vi "matrix.vi"(2 "B":T2, 3 "A":T3) -> (0 "P":T1, 1 "X0":bool)   [LabVIEW 2013]
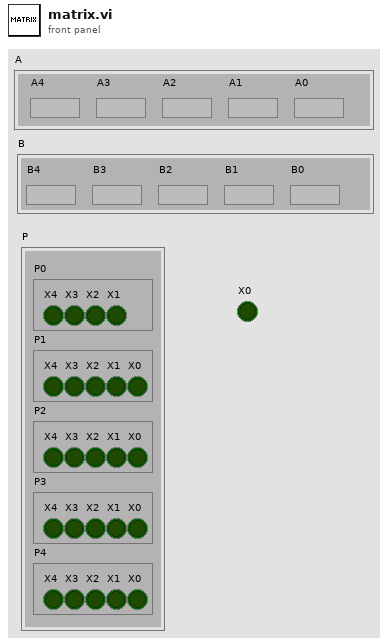
[diagram p1: front panel]
types:
  T1 = cluster{"P0":cluster{"X4":bool, "X3":bool, "X2":bool, "X1":bool}, "P1":cluster{"X4":bool, "X3":bool, "X2":bool, "X1":bool, "X0":bool}, "P2":cluster{"X4":bool, "X3":bool, "X2":bool, "X1":bool, "X0":bool}, "P3":cluster{"X4":bool, "X3":bool, "X2":bool, "X1":bool, "X0":bool}, "P4":cluster{"X4":bool, "X3":bool, "X2":bool, "X1":bool, "X0":bool}}
  T2 = cluster{"B4":bool, "B3":bool, "B2":bool, "B1":bool, "B0":bool}
  T3 = cluster{"A4":bool, "A3":bool, "A2":bool, "A1":bool, "A0":bool}
  T4 = cluster{cluster{bool, bool, bool, bool}, cluster{bool, bool, bool, bool, bool}, cluster{bool, bool, bool, bool, bool}, cluster{bool, bool, bool, bool, bool}, cluster{bool, bool, bool, bool, bool}}
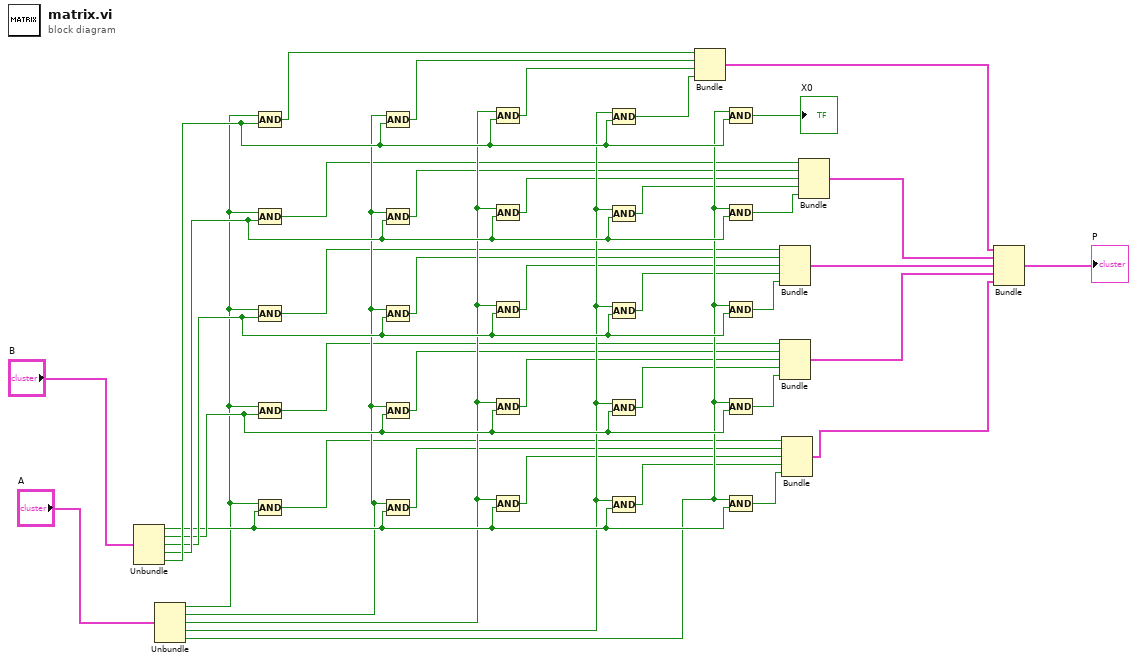
[diagram p0: block diagram]
diagram:
  n1 = Unbundle("B") -> ("B4"=w37:bool, "B3"=w38:bool, "B2"=w39:bool, "B1"=w40:bool, "B0"=w41:bool)
  n2 = Unbundle("A") -> ("A4"=w32:bool, "A3"=w33:bool, "A2"=w34:bool, "A1"=w35:bool, "A0"=w36:bool)
  n3 = Compound Arithmetic op=AND(w32, w41) -> (w27:bool)
  n4 = Compound Arithmetic op=AND(w32, w40) -> (w22:bool)
  n5 = Compound Arithmetic op=AND(w32, w39) -> (w17:bool)
  n6 = Compound Arithmetic op=AND(w32, w38) -> (w12:bool)
  n7 = Compound Arithmetic op=AND(w32, w37) -> (w7:bool)
  n8 = Compound Arithmetic op=AND(w33, w41) -> (w28:bool)
  n9 = Compound Arithmetic op=AND(w33, w40) -> (w23:bool)
  n10 = Compound Arithmetic op=AND(w33, w39) -> (w18:bool)
  n11 = Compound Arithmetic op=AND(w33, w38) -> (w13:bool)
  n12 = Compound Arithmetic op=AND(w33, w37) -> (w8:bool)
  n13 = Compound Arithmetic op=AND(w34, w41) -> (w29:bool)
  n14 = Compound Arithmetic op=AND(w34, w40) -> (w24:bool)
  n15 = Compound Arithmetic op=AND(w34, w39) -> (w19:bool)
  n16 = Compound Arithmetic op=AND(w34, w38) -> (w14:bool)
  n17 = Compound Arithmetic op=AND(w34, w37) -> (w9:bool)
  n18 = Compound Arithmetic op=AND(w35, w41) -> (w30:bool)
  n19 = Compound Arithmetic op=AND(w35, w40) -> (w25:bool)
  n20 = Compound Arithmetic op=AND(w35, w39) -> (w20:bool)
  n21 = Compound Arithmetic op=AND(w35, w38) -> (w15:bool)
  n22 = Compound Arithmetic op=AND(w35, w37) -> (w10:bool)
  n23 = Bundle(w27, w28, w29, w30) -> (w5:cluster{bool, bool, bool, bool})  [unwired: 1 in]
  n24 = Compound Arithmetic op=AND(w36, w41) -> (→"X0":bool)
  n25 = Compound Arithmetic op=AND(w36, w40) -> (w26:bool)
  n26 = Compound Arithmetic op=AND(w36, w39) -> (w21:bool)
  n27 = Compound Arithmetic op=AND(w36, w38) -> (w16:bool)
  n28 = Compound Arithmetic op=AND(w36, w37) -> (w11:bool)
  n29 = Bundle(w17, w18, w19, w20, w21) -> (w3:cluster{bool, bool, bool, bool, bool})  [unwired: 1 in]
  n30 = Bundle(w12, w13, w14, w15, w16) -> (w2:cluster{bool, bool, bool, bool, bool})  [unwired: 1 in]
  n31 = Bundle(w7, w8, w9, w10, w11) -> (w1:cluster{bool, bool, bool, bool, bool})  [unwired: 1 in]
  n32 = Bundle(w22, w23, w24, w25, w26) -> (w4:cluster{bool, bool, bool, bool, bool})  [unwired: 1 in]
  n33 = Bundle(w5, w4, w3, w2, w1) -> (→"P":T4)  [unwired: 1 in]
